vi "Write RemIO Module Page Property.vi"(8 "error in (no error)":errorcluster, 10 "Node Ptr In":T1 format="%.0x", 11 "RemIO Module":refnum<class "RemIO Module.lvclass">) -> (0 "error out":errorcluster, 2 "Node Ptr Out":T1 format="%.0x", 3 "RemIO Module Out":refnum<class "RemIO Module.lvclass">)   [LabVIEW 2020, in "Modules.lvlib" / "RemIO Module.lvclass"]
uses:
  RemIO Module.lvclass
  <vilib>/NI VeriStand/Custom Device API/Custom Device Item Ref.ctl
  RSI Module/Class Property Strings.vi
  <vilib>/NI VeriStand/Custom Device API/Set Item Property (String).vi
  <vilib>/NI VeriStand/Custom Device API/Custom Device API.lvlib
  RSI Module/RSI Module.lvclass
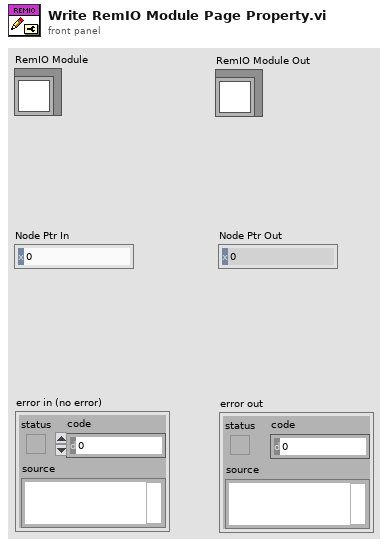
[diagram p1: front panel]
types:
  T1 = typedef "Custom Device API.lvlib/Custom Device Item Ref.ctl" = u64
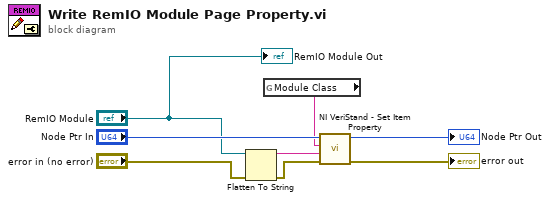
[diagram p0: block diagram]
diagram:
  n1 = Flatten To String(anything="RemIO Module", error in (no error)="error in (no error)") -> (data string=w4:string, error out=w3:errorcluster)  [unwired: 2 in, 1 out]
  n2 = global read "Class Property Strings.vi" "Module Class"() -> (w2:string)
  n3 = call-poly <vilib>:"NI VeriStand - Set Item Property.vi"("error in (no error)"=w3, "Value"=w4, "Property Name"=w2, "Item Ref in"="Node Ptr In") -> ("error out"=→"error out":errorcluster, "Item Ref out"=→"Node Ptr Out":T1)  [unwired: 5 in, 1 out]
  "RemIO Module Out" <- "RemIO Module"
